vi "HSDIO_6541_Script_Loader.vi"(3 "error in (no error)":errorcluster, 4 "instrument handle in":refnum<k15> caption="instrument handle") -> (0 "error out":errorcluster, 1 "instrument handle out":refnum<k15>)   [LabVIEW 2015]
doc: "Load one or more scripts into the on-board FIFO that govern the generation of waveforms. \nCAUTION : waveforms must be loaded BEFORE the scripts."
panel:
  in  "Script text":string
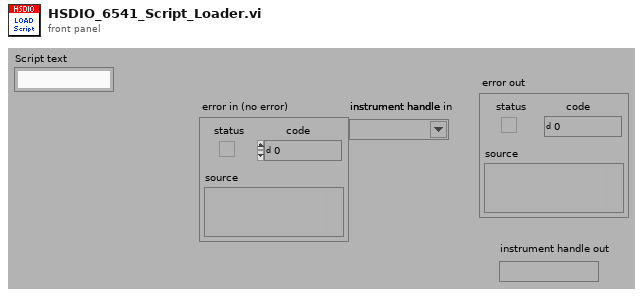
[diagram p1: front panel]
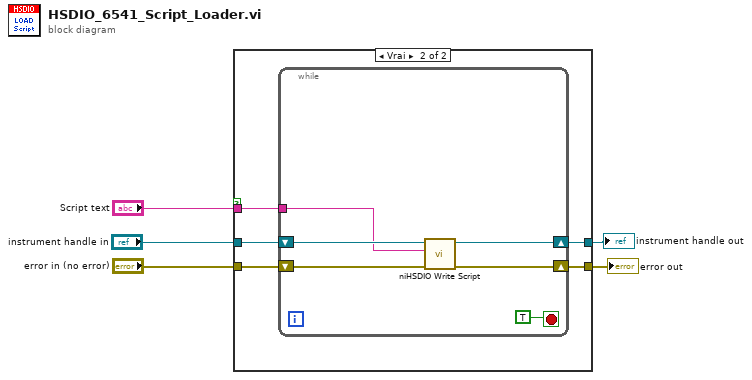
[diagram p0: block diagram]
diagram:
  n1 = case shown="Vrai" {
    selector: _ -> [_ _]
    tunnel: "error in (no error)" -> [_ w10]
    tunnel: "instrument handle in" -> [_ w9]
    tunnel: [_ w8] -> w3
    tunnel: [_ w7] -> w2
    tunnel: "Script text" -> [_ w6]
    frame False {
    }
    frame True {
      n2 = while {
        shift-right: [w13] -> w7
        shift-left: w10 -> [w16]
        shift-right: [w14] -> w8
        shift-left: w9 -> [w15]
        tunnel: w6 -> [w11]
        stop <- TRUE stop-if-true
        n3 = call <instrlib>:"niHSDIO Write Script.vi"("error in (no error)"=w16, "script"=w11, "instrument handle"=w15) -> ("error out"=w13:errorcluster, "instrument handle out"=w14:refnum<k15>)  [unwired: 7 in]
      }
    }
  }
  "instrument handle out" <- w3
  "error out" <- w2
